vi "Configure Frequency.vi"(0 "VISA resource name":refnum<visa-resource-name>, 5 "Output AC Voltage Frequency (60  Hz)":dbl=60.0 min=45.0 max=500.0 format="%.1p", 11 "error in (no error)":errorcluster) -> (4 "VISA resource name out":refnum<visa-resource-name>, 15 "error out":errorcluster)   [LabVIEW 2020, in "eec 6700.lvlib"]
doc: "Sets <B>Frequency</B> of the output in the power source instrument.\n\nThe value should be in the configured Test limit\n\nIt is the number of times a waveform completes a cycle in a period of time."
uses:
  <instrlib>/EEC6700LV-driver/eec 6700.lvlib
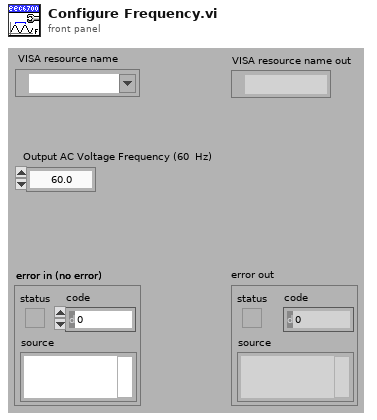
[diagram p1: front panel]
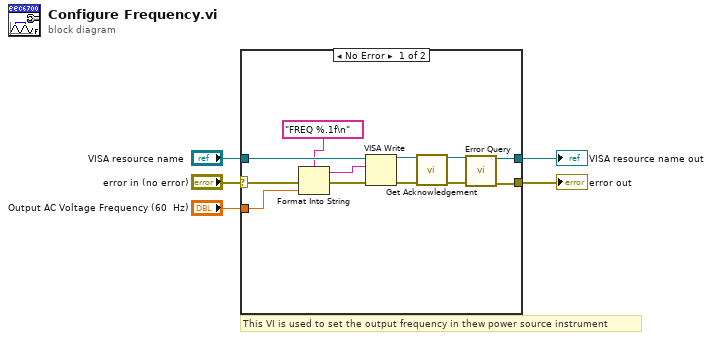
[diagram p0: block diagram]
diagram:
  # "This VI is used to set the output frequency in thew power source instrument"
  n1 = case shown="No Error" "error in (no error)" {
    selector: "error in (no error)" -> [w11 w19]
    tunnel: [w12 w19] -> w5
    tunnel: [w13 w18] -> w4
    tunnel: "VISA resource name" -> [w17 w18]
    tunnel: "Output AC Voltage Frequency (60  Hz)" -> [w16 _]
    frame No Error {
      n2 = Format Into String(format string="FREQ %.1f\n" ("Command"), error in=w11, w16) -> (resulting string=w15:string, error out=w10:errorcluster)  [unwired: 1 in]
      n3 = VISA Write(VISA resource name=w17, write buffer=w15, error in (no error)=w10) -> (VISA resource name out=w7:refnum<visa-resource-name>, error out=w6:errorcluster)  [unwired: 1 out]
      n4 = call <instrlib>:"Get Acknowledgement.vi"("VISA resource name"=w7, "error in (no error)"=w6) -> ("VISA resource name out"=w8:refnum<visa-resource-name>, "error out"=w9:errorcluster)  [unwired: 12 in]
      n5 = call <instrlib>:"Error Query.vi"("VISA resource name"=w8, "error in (no error)"=w9) -> ("VISA resource name out"=w13:refnum<visa-resource-name>, "error out"=w12:errorcluster)  [unwired: 10 in, 2 out]
    }
    frame Error {
    }
  }
  "error out" <- w5
  "VISA resource name out" <- w4
